vi "Get Test Result Filename.vi"() -> (0 "TestResult Filename out":string)   [LabVIEW 2017]
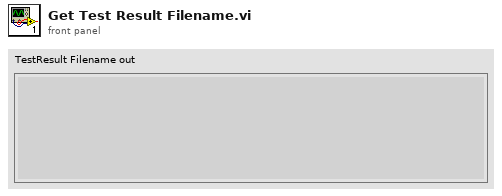
[diagram p1: front panel]
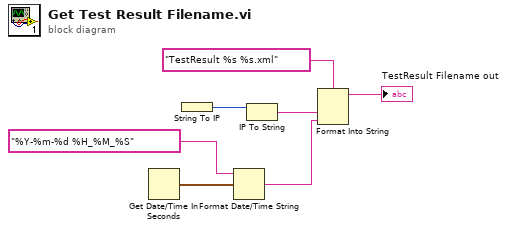
[diagram p0: block diagram]
diagram:
  n1 = Get Date/Time In Seconds() -> (seconds since 1Jan1904=w4:timestamp)
  n2 = String To IP() -> (0:w7:u32)  [unwired: 1 in]
  n3 = Format Date/Time String(time format string (%c)="%Y-%m-%d %H_%M_%S", seconds (now)=w4) -> (date/time string=w3:string)  [unwired: 1 in]
  n4 = IP To String(2:w7) -> (0:w5:string)  [unwired: 1 in]
  n5 = Format Into String(format string="TestResult %s %s.xml", w5, w3) -> (resulting string=→"TestResult Filename out":string)  [unwired: 2 in, 1 out]
